vi "2023_day06.vi"() -> ()   [LabVIEW 2021]
panel:
  out "Task 2":i32
  out "Task 1":i32
  in  "Switch":bool caption="Ex. Data  vs.  User Data"
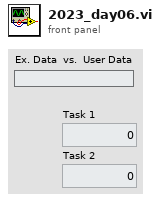
[diagram p1: front panel]
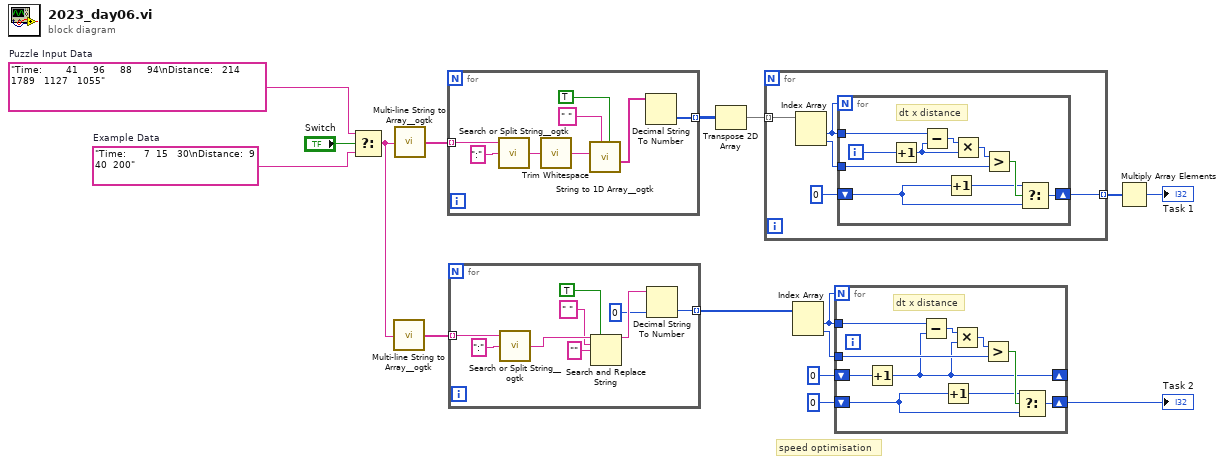
[diagram p0: block diagram]
diagram:
  w15 = "Time:        41     96     88     94\nDistance:   214   1789   1127   1055"  # Puzzle Input Data
  w10 = "Time:      7  15   30\nDistance:  9  40  200"  # Example Data
  # "speed optimisation"
  n1 = Select(t=w15, s="Switch", f=w10) -> (s? t:f=w6:string)
  n2 = call <userlib>:"Multi-line String to Array__ogtk.vi"("string"=w6) -> ("lines"=w11:string[])
  n3 = call <userlib>:"Multi-line String to Array__ogtk.vi"("string"=w6) -> ("lines"=w14:string[])
  n4 = for {
    tunnel: w14 -> [w24] mode=indexing
    tunnel: [w17] -> w13 mode=indexing
    n5 = call <userlib>:"Search or Split String__ogtk.vi"("search string/char (-)"=":", "string"=w24) -> ("substring after match"=w22:string)  [unwired: 1 in, 2 out]
    n6 = call <vilib>:"Trim Whitespace.vi"("string"=w22) -> ("trimmed string"=w18:string)  [unwired: 1 in]
    n7 = call <userlib>:"String to 1D Array__ogtk.vi"("ignore duplicate delimiters? (F=No)"=TRUE, "delimiter (Tab)"=" ", "string"=w18) -> ("Array of Strings"=w19:string[])  [unwired: 8 in]
    n8 = Decimal String To Number(string=w19) -> (number=w17:i32[])  [unwired: 2 in, 1 out]
  }
  n9 = for {
    tunnel: w11 -> [w33] mode=indexing
    tunnel: [w31] -> w9 mode=indexing
    n10 = call <userlib>:"Search or Split String__ogtk.vi"("search string/char (-)"=":", "string"=w33) -> ("substring after match"=w29:string)  [unwired: 1 in, 2 out]
    n11 = Search and Replace String(replace all?=TRUE ("ignore duplicate delimiters? (F=No)"), input string=w29, search string=" " ("delimiter (Tab)"), replace string="" ("replace string (\"\")")) -> (result string=w26:string)  [unwired: 4 in, 3 out]
    n12 = Decimal String To Number(string=w26, default (0L)=u64 0 ("default (0 I32)")) -> (number=w31:u64)  [unwired: 1 in, 1 out]
  }
  n13 = Transpose 2D Array(2D array=w13) -> (transposed array=w12:i32[][])
  n14 = for {
    tunnel: w12 -> [w35] mode=indexing
    tunnel: [w34] -> w3 mode=indexing
    n15 = Index Array(array=w35) -> (element #1=w37:i32, element #2=w38:i32)  [unwired: 2 in]
    n16 = for {
      N: w37 -> [_]
      tunnel: w37 -> [w46]
      tunnel: w38 -> [w44]
      shift-right: [w42] -> w34
      shift-left: 0 -> [w39]
      i -> [w48]
      # "dt x distance"
      n17 = Increment(x=w48) -> (x+1=w45:i32)
      n18 = Subtract(x=w46, y=w45) -> (x-y=w47:i32)
      n19 = Increment(x=w39) -> (x+1=w40:i32)
      n20 = Multiply(x=w47, y=w45) -> (x*y=w43:i32)
      n21 = Greater?(x=w43, y=w44) -> (0:w41:bool)
      n22 = Select(t=w40, s=w41, f=w39) -> (s? t:f=w42:i32)
    }
  }
  n23 = Index Array(array=w9) -> (element #1=w7:u64, element #2=w8:u64)  [unwired: 2 in]
  n24 = for {
    N: w7 -> [_]
    tunnel: w7 -> [w57]
    tunnel: w8 -> [w56]
    shift-right: [w54] -> w4
    shift-left: 0 -> [w51]
    shift-right: [w49] -> _
    shift-left: u64 0 -> [w50]
    # "dt x distance"
    n25 = Increment(x=w50) -> (x+1=w49:u64)
    n26 = Subtract(x=w57, y=w49) -> (x-y=w58:u64)
    n27 = Increment(x=w51) -> (x+1=w52:i32)
    n28 = Multiply(x=w58, y=w49) -> (x*y=w55:u64)
    n29 = Greater?(x=w55, y=w56) -> (0:w53:bool)
    n30 = Select(t=w52, s=w53, f=w51) -> (s? t:f=w54:i32)
  }
  "Task 2" <- w4
  n31 = Multiply Array Elements(1:w3) -> (0:→"Task 1":i32)
